vi "Tester 1.vi"() -> ()   [LabVIEW 2016, in "Error Manager.lvlib" / "Error Display Window.lvclass"]
doc: "Tester 1"
uses:
  Error Display Window.lvclass
  Error Details (cluster).ctl
panel:
  out "Error Out":errorcluster
  # "Tester 1"
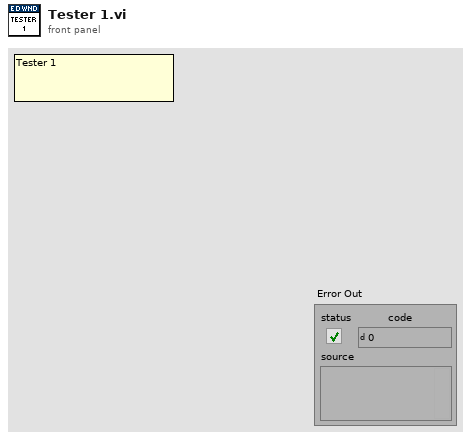
[diagram p1: front panel]
types:
  T1 = typedef "Error Manager.lvlib/Error Display Window.lvclass/Error Details (cluster).ctl" = cluster{"Error Code":i32, "Error Message":string, "Error Timestamp":timestamp}
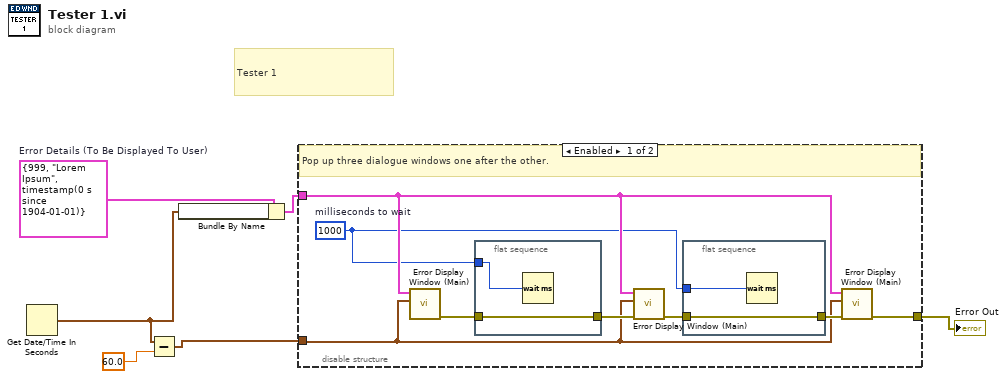
[diagram p0: block diagram]
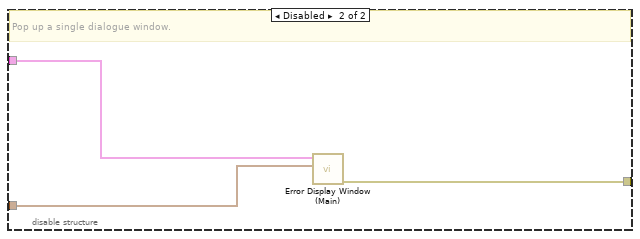
[diagram p2: hidden frame]
diagram:
  w5 = T1 {"Error Code"=999, "Error Message"="Lorem Ipsum", "Error Timestamp"=timestamp(0 s since 1904-01-01)}  # Error Details (To Be Displayed To User)
  # "Tester 1"
  n1 = Get Date/Time In Seconds() -> (seconds since 1Jan1904=w3:timestamp)
  n2 = Subtract(x=w3, y=60.0) -> (x-y=w1:timestamp)
  n3 = Bundle By Name(cluster=w5, w3) -> (w4:T1)
  n4 = disable-structure shown="Enabled" {
    disable-tunnel: [w10 w21] -> w6
    disable-tunnel: w4 -> [w9 w20]
    disable-tunnel: w1 -> [w8 w19]
    frame Enabled {
      w7 = u32 1000  # milliseconds to wait
      # "Pop up three dialogue windows one after the other."
      n5 = call "Error Display Window (Main).vi"(10:w8, 11:w9) -> (0:w14:errorcluster)  [unwired: 9 in]
      n6 = flat-sequence {
        tunnel: w14 -> [w16]
        tunnel: [w16] -> w12
        tunnel: w7 -> [w15]
        frame #0 {
          n7 = Wait (ms)(milliseconds to wait=w15) -> ()  [unwired: 1 out]
        }
      }
      n8 = call "Error Display Window (Main).vi"(8:w12, 10:w8, 11:w9) -> (0:w13:errorcluster)  [unwired: 8 in]
      n9 = flat-sequence {
        tunnel: w13 -> [w18]
        tunnel: [w18] -> w11
        tunnel: w7 -> [w17]
        frame #0 {
          n10 = Wait (ms)(milliseconds to wait=w17) -> ()  [unwired: 1 out]
        }
      }
      n11 = call "Error Display Window (Main).vi"(8:w11, 10:w8, 11:w9) -> (0:w10:errorcluster)  [unwired: 8 in]
    }
    frame Disabled {
      # "Pop up a single dialogue window."
      n12 = call "Error Display Window (Main).vi"(10:w19, 11:w20) -> (0:w21:errorcluster)  [unwired: 9 in]
    }
  }
  "Error Out" <- w6
